vi "FRCts20_Backend_Team_GETIndex.vi"(6 "Message Attributes":T4, 8 "error in (no error)":errorcluster, 10 "Data":string, 11 "Engine_Refnums":T1) -> (0 "error out":errorcluster)   [LabVIEW 2014, in "FRCts20_Backend_Engine.lvlib"]
doc: "Gets all information and requests under a selected team. Called by the Team API, expects a team index"
uses:
  FRCts20_Backend_Engine.lvlib
  Dependencies/Keyed Array/KeyedArray.ctl
  FRCts20_Backend_EngineRefnums.ctl
  INI_Accessor/FRCts20_Backend_INI Controller.lvclass
  Dependencies/AMC/_SubVIs/TypeDefs/Message Queue.ctl
  Dependencies/AMC/_SubVIs/TypeDefs/Message.ctl
  <vilib>/addons/database/Connection.llb/Conn ObjectReference.ctl
  FRCts20_Backend_API/FRCts20_Backend_API_Team.ctl
  FRCts20_Backend_API/FRCts20_Backend_API_SW.ctl
  FRCts20_Backend_API/FRCts20_Backend_API_Status.ctl
  FRCts20_Backend_FGVOperation.ctl
  FRCts20_Backend_API/FRCts20_Backend_API.lvlib
  Dependencies/Keyed Array/Tools_KeyedArray.lvlib
  Dependencies/AMC/AMC.lvlib
  <vilib>/addons/database/NI_Database_API.lvlib
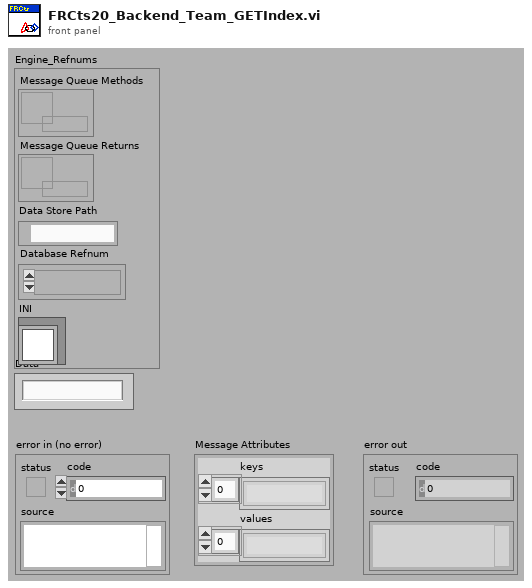
[diagram p1: front panel]
types:
  T1 = typedef "FRCts20_Backend_Engine.lvlib/FRCts20_Backend_EngineRefnums.ctl" = cluster{"Message Queue Methods":T2, "Message Queue Returns":T2, "Data Store Path":path, "Database Refnum":T3, "INI":refnum<class "FRCts20_Backend_INI Controller.lvclass">}
  T2 = typedef "AMC.lvlib/Message Queue.ctl" = refnum<queue>
  T3 = typedef "NI_Database_API.lvlib/Conn ObjectReference.ctl" = refnum<k1>
  T4 = typedef "Tools_KeyedArray.lvlib/KeyedArray.ctl" = cluster{"keys":string[], "values":string[]}
  T5 = typedef "FRCts20_Backend_Engine.lvlib/FRCts20_Backend_FGVOperation.ctl" = enum16{"Initialize", "EnqueueMessage", "EnqueueDataReturn", "FlushMessage", "FlushDataReturn"}
  T6 = typedef "FRCts20_Backend_Engine.lvlib/FRCts20_Backend_API.lvlib/FRCts20_Backend_API_Team.ctl" = cluster{"Team Index":u32, "Team Number":u32, "Team Name":string, "Short Team Name":string, "Nick Name":string, "Robot Name":string, "City":string, "State":string, "Country":string, "Rookie Year":u32, "SWType":T7, "CAN":bool, "Vision":bool, "Kinect":bool, "Tags":string, "Avatar":string, "Request Array":cluster{"Request Index":u32, "Description":string, "Status":T8, "Open Date":timestamp, "Last Update":timestamp, "Close Date":timestamp}[], "Events Attending":cluster{"EventIndex":dbl, "EventName":string, "IsLive":bool}[], "APIReturn":string}
  T7 = typedef "FRCts20_Backend_Engine.lvlib/FRCts20_Backend_API.lvlib/FRCts20_Backend_API_SW.ctl" = string
  T8 = typedef "FRCts20_Backend_Engine.lvlib/FRCts20_Backend_API.lvlib/FRCts20_Backend_API_Status.ctl" = enum16{"Open", "In Work", "Closed"}
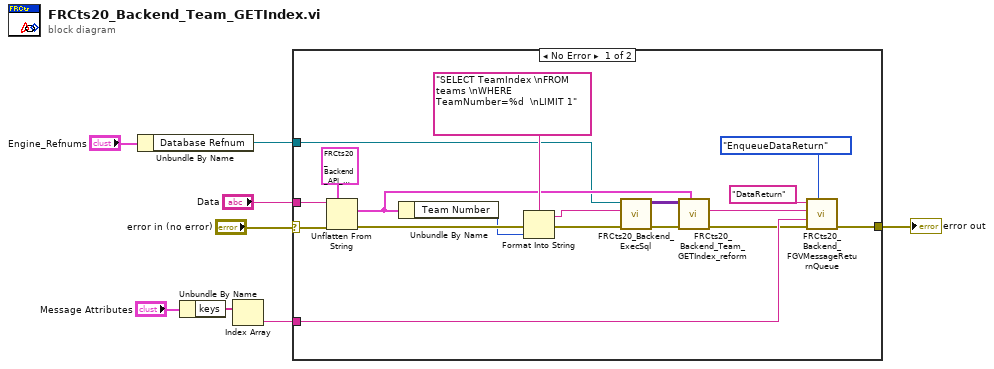
[diagram p0: block diagram]
diagram:
  n1 = Unbundle By Name("Engine_Refnums") -> ("Database Refnum"=w1:T3)
  n2 = Unbundle By Name("Message Attributes") -> ("keys"=w4:string[])
  n3 = Index Array(array=w4) -> (element=w3:string)  [unwired: 1 in]
  n4 = case shown="No Error" "error in (no error)" {
    selector: "error in (no error)" -> [w23 w27]
    tunnel: [w26 w27] -> w7
    tunnel: w1 -> [w12 _]
    tunnel: "Data" -> [w24 _]
    tunnel: w3 -> [w25 _]
    frame No Error {
      n5 = Unflatten From String(type=T6 {"Team Index"=0, "Team Number"=0, "Team Name"="", "Short Team Name"="", "Nick Name"="", "Robot Name"="", "City"="", "State"="", "Country"="", "Rookie Year"=0, "SWType"="", "CAN"=FALSE, "Vision"=FALSE, "Kinect"=FALSE, "Tags"="", "Avatar"="", "Request Array"=[], "Events Attending"=[], "APIReturn"=""} ("Team"), binary string=w24, error in (no error)=w23) -> (value=w13:T6, error out=w11:errorcluster)  [unwired: 2 in, 1 out]
      n6 = Unbundle By Name(w13) -> ("Team Number"=w10:u32)
      n7 = Format Into String(format string="SELECT TeamIndex \nFROM teams \nWHERE TeamNumber=%d  \nLIMIT 1", error in=w11, w10) -> (resulting string=w14:string, error out=w16:errorcluster)  [unwired: 1 in]
      n8 = call "FRCts20_Backend_ExecSql.vi"("error in (no error)"=w16, "format string"=w14, "Refnum in"=w12) -> ("error out"=w9:errorcluster, "recordset data"=w15:variant[][])  [unwired: 6 in, 1 out]
      n9 = call "FRCts20_Backend_Team_GETIndex_reform.vi"("Team"=w13, "error in (no error)"=w9, "teamdata"=w15) -> ("error out"=w21:errorcluster, "data string"=w18:string)  [unwired: 7 in]
      n10 = call "FRCts20_Backend_FGVMessageReturnQueue.vi"("Operation"=FRCts20_Backend_FGVOperation."EnqueueDataReturn", "error in (no error)"=w21, "Key"=w25, "Message Value"=w18, "Message Name"="DataReturn") -> ("error out"=w26:errorcluster)  [unwired: 5 in, 1 out]
    }
    frame Error {
    }
  }
  "error out" <- w7
